vi "Read.vi"(8 "error in (no error)":errorcluster, 11 "Notifiers in":refnum<class "Notifiers.lvclass">) -> (0 "error out":errorcluster, 2 "DATA":T1, 3 "Notifiers out":refnum<class "Notifiers.lvclass">)   [LabVIEW 2020, in "Notifiers.lvclass"]
uses:
  Notifiers.lvclass
  Notifiers.lvclass/Notifiers.ctl
  Accessors/Read/Read DATA_Notifiers.vi
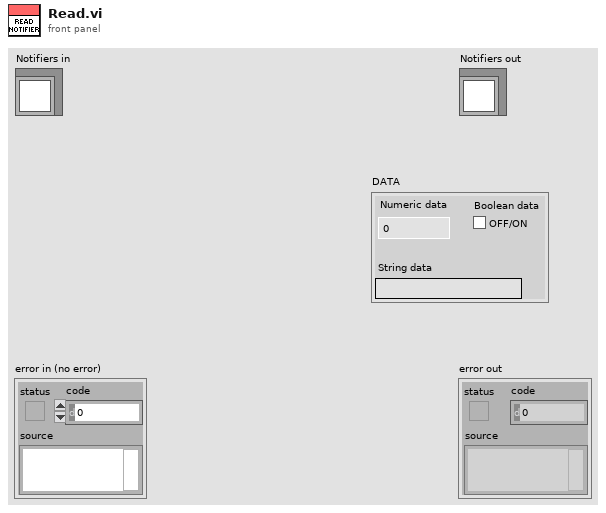
[diagram p1: front panel]
types:
  T1 = cluster{"Numeric data":dbl, "String data":string, "Boolean data":bool}
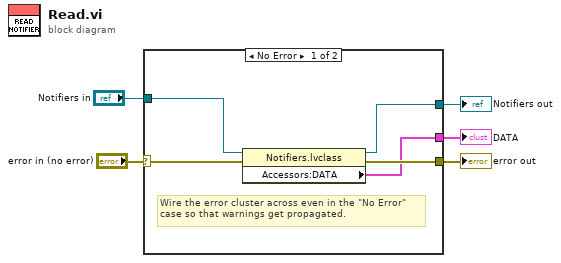
[diagram p0: block diagram]
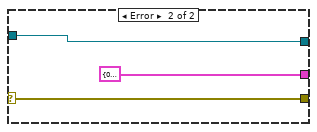
[diagram p2: hidden frame]
diagram:
  n1 = case shown="No Error" "error in (no error)" {
    selector: "error in (no error)" -> [w10 w13]
    tunnel: [w9 w13] -> w4
    tunnel: [w6 w12] -> w2
    tunnel: "Notifiers in" -> [w8 w12]
    tunnel: [w7 T1 {"Numeric data"=0.0, "String data"="", "Boolean data"=FALSE} ("Accessors:DATA")] -> w1
    frame No Error {
      # "Wire the error cluster across even in the \"No Error\"\ncase so that warnings get propagated."
      n2 = property class="Notifiers.lvclass"(reference=w8, error in=w10) -> (reference out=w6:refnum<class "Notifiers.lvclass">, error out=w9:errorcluster, "Accessors:DATA"=w7:T1)
    }
    frame Error {
    }
  }
  "error out" <- w4
  "Notifiers out" <- w2
  "DATA" <- w1
